vi "Untitled 1.vi"() -> (1 "created new?":bool, 3 "queue out":refnum<queue>)   [LabVIEW 2017, in "MDPtr.lvlib"]
uses:
  MDPtr.lvlib
  MDPtr TypeDef/MDPtr.ctl
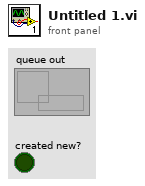
[diagram p1: front panel]
types:
  T1 = typedef "MDPtr.lvlib/MDPtr.ctl" = refnum<k1>
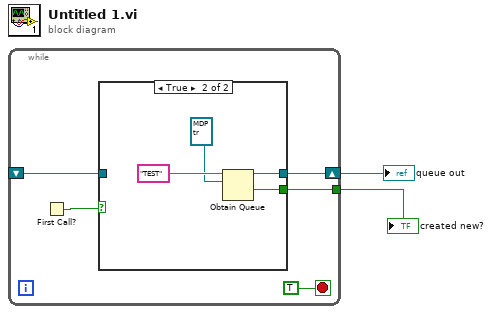
[diagram p0: block diagram]
diagram:
  n1 = while {
    shift-right: [w5] -> w2
    shift-left: _ -> [w4]
    tunnel: [w3] -> w1
    stop <- TRUE stop-if-true
    n2 = First Call?() -> (First Call?: T/F=w6:bool)
    n3 = case shown="True" w6 {
      tunnel: [w8 w11] -> w5
      tunnel: w4 -> [w8 _]
      tunnel: [_ w9] -> w3
      frame False {
      }
      frame True {
        n4 = Obtain Queue(name (unnamed)="TEST", element data type=T1 refnum ("MDPtr")) -> (queue out=w11:refnum<queue>, created new?=w9:bool)  [unwired: 3 in, 1 out]
      }
    }
  }
  "queue out" <- w2
  "created new?" <- w1
